vi "Read Range.vi"(8 "error in (no error)":errorcluster, 11 "DAQ Configuration in":refnum<class "DAQ Configuration.lvclass">) -> (0 "error out":errorcluster, 2 "Range":cluster{"Ranve (min)":dbl, "Range Max":dbl}, 3 "DAQ Configuration out":refnum<class "DAQ Configuration.lvclass">)   [LabVIEW 2017, in "Hardware.lvlib" / "DAQ Configuration.lvclass"]
uses:
  DAQ Configuration.lvclass
  DAQ Configuration.lvclass/DAQ Configuration.ctl
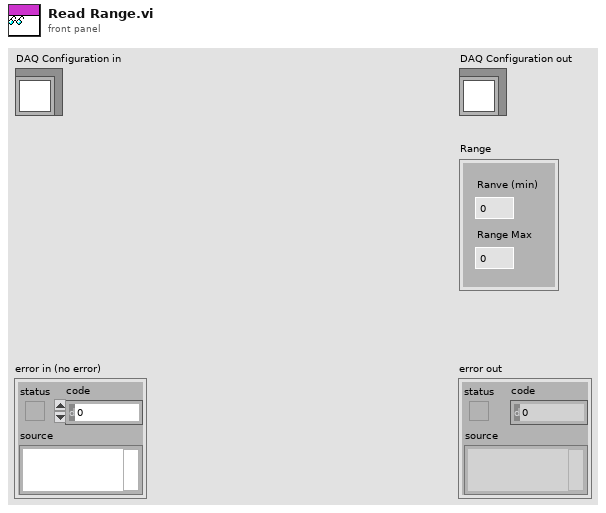
[diagram p1: front panel]
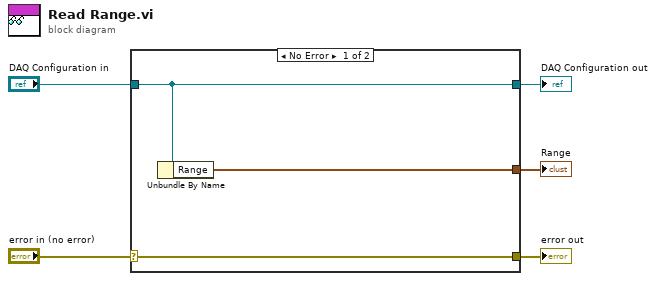
[diagram p0: block diagram]
diagram:
  n1 = case shown="No Error" "error in (no error)" {
    selector: "error in (no error)" -> [w8 w9]
    tunnel: [w8 w9] -> w4
    tunnel: [w7 w10] -> w2
    tunnel: "DAQ Configuration in" -> [w7 w10]
    tunnel: [w6 _] -> w1
    frame No Error {
      n2 = Unbundle By Name(w7) -> ("Range"=w6:cluster{"Ranve (min)":dbl, "Range Max":dbl})
    }
    frame Error {
    }
  }
  "error out" <- w4
  "DAQ Configuration out" <- w2
  "Range" <- w1
